vi "ValveFGV.vi"(8 "Valve Data":T1, 9 "ignore previous (F)":bool, 10 "timeout in ms (-1)":i32=-1, 11 "Action":T2(ring)=enum."Create") -> (0 "error out":errorcluster, 1 "Valve Data Out":T1, 2 "timed out?":bool=TRUE, 5 "queue out":refnum<queue>)   [LabVIEW 2016]
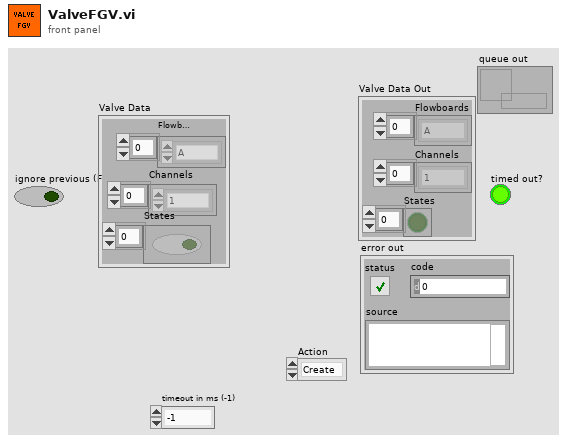
[diagram p1: front panel]
types:
  T1 = cluster{"Flowboards":enum16{"A", "B", "C"}[], "Channels":enum16{"1", "2", "3", "4", "5", "6", "7", "8"}[], "States":bool[]}
  T2 = enum16{"Release", "Create", "Send", "Wait", "Cancel"}
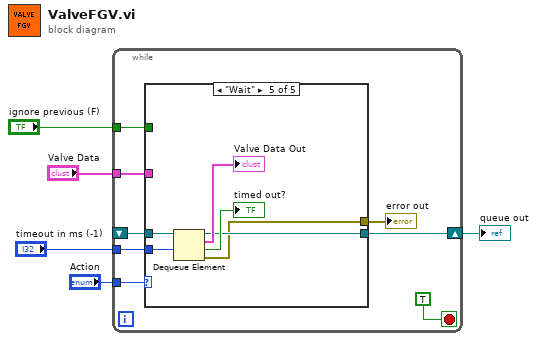
[diagram p0: block diagram]
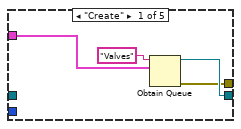
[diagram p2: hidden frame]
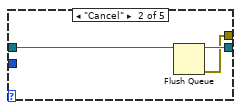
[diagram p3: hidden frame]
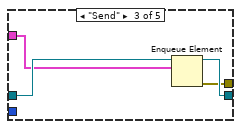
[diagram p4: hidden frame]
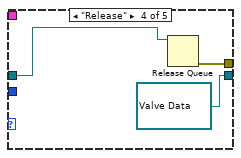
[diagram p5: hidden frame]
diagram:
  n1 = while {
    tunnel: "Action" -> [w13]
    shift-right: [w12] -> w1
    shift-left: _ -> [w11]
    tunnel: "timeout in ms (-1)" -> [w10]
    tunnel: "ignore previous (F)" -> [w8]
    tunnel: "Valve Data" -> [w7]
    stop <- TRUE stop-if-true
    n2 = case shown="\"Wait\"" w13 {
      tunnel: [w16 w19 w23 refnum<queue> refnum ("queue out") w29] -> w12
      tunnel: w11 -> [_ w20 w24 w25 w33]
      tunnel: w10 -> [_ _ _ _ w32]
      tunnel: w8 -> [_ _ _ _ _]
      tunnel: w7 -> [w15 _ w21 _ _]
      tunnel: [w14 w18 w22 w26 w28] -> w6
      frame "Create" {
        n3 = Obtain Queue(name (unnamed)="Valves", element data type=w15) -> (queue out=w16:refnum<queue>, error out=w14:errorcluster)  [unwired: 3 in, 1 out]
      }
      frame "Cancel" {
        n4 = Flush Queue(queue=w20) -> (queue out=w19:refnum<queue>, error out=w18:errorcluster)  [unwired: 1 in, 1 out]
      }
      frame "Send" {
        n5 = Enqueue Element(queue=w24, element=w21) -> (queue out=w23:refnum<queue>, error out=w22:errorcluster)  [unwired: 2 in, 1 out]
      }
      frame "Release" {
        n6 = Release Queue(queue=w25) -> (error out=w26:errorcluster)  [unwired: 2 in, 2 out]
      }
      frame "Wait" {
        n7 = Dequeue Element(queue=w33, timeout in ms (-1)=w32) -> (queue out=w29:refnum<queue>, element=→"Valve Data Out":T1, timed out?=→"timed out?":bool, error out=w28:errorcluster)  [unwired: 1 in]
      }
    }
    "error out" <- w6
  }
  "queue out" <- w1
